vi "Untitled_1.vi"() -> ()   [LabVIEW 2018]
panel:
  in  "Cluster":cluster{"OK Button":bool}
  in  "Array":bool[](array[boolean])
  in  "stop":bool
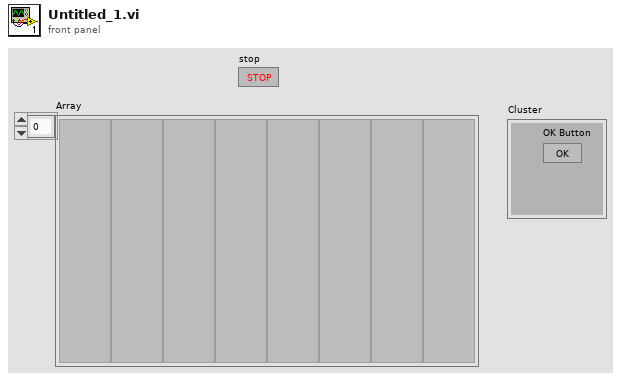
[diagram p1: front panel]
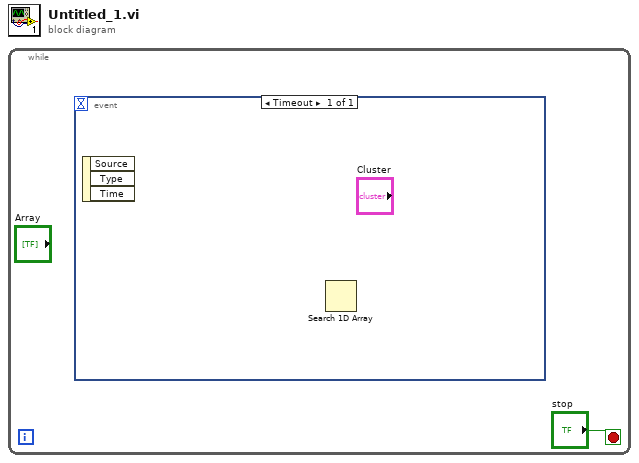
[diagram p0: block diagram]
diagram:
  n1 = while {
    stop <- "stop" stop-if-true
    n2 = event shown="[0] Timeout" {
      selector: _ -> [_]
      dyn-events: _ -> [_]
      timeout: _ -> [_]
      event Timeout {
        n3 = event-data() -> ()  [unwired: 1 in, 3 out]
        n4 = Search 1D Array() -> ()  [unwired: 3 in, 1 out]
      }
    }
  }
